vi "ADCReq.vi"(0 "aDATA":u8[](array[numeric]), 4 "Gain":dbl, 5 "Rsense":dbl) -> (12 "NumOut 1":dbl)   [LabVIEW 2010]
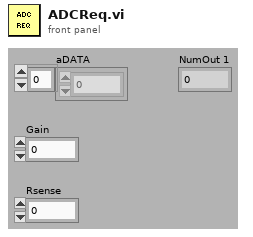
[diagram p1: front panel]
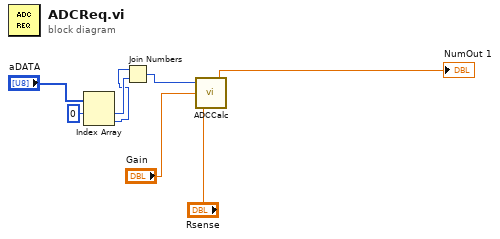
[diagram p0: block diagram]
diagram:
  n1 = Index Array(array="aDATA", index #1=0 ("index")) -> (element #1=w3:u8, element #2=w2:u8)  [unwired: 1 in]
  n2 = Join Numbers(hi=w2, lo=w3) -> ((hi.lo)=w1:u16)
  n3 = call "ADCCalc.vi"("Rsense"="Rsense", "Gain"="Gain", "DATA"=w1) -> ("NumOut"=→"NumOut 1":dbl)
